vi "Routing Channels.vi"(8 "error in (no error)":errorcluster, 11 "Node Ptr":T1 format="%.0x") -> (0 "error out":errorcluster)   [LabVIEW 2017, in "Routing and Faulting System Explorer.lvlib"]
uses:
  Routing and Faulting System Explorer.lvlib
  <vilib>/NI Veristand/Custom Device API/Custom Device Item Ref.ctl
  Main Page Controls.ctl
  <vilib>/NI VeriStand/Custom Device API/Custom Device API.lvlib
panel:
  out "Version":string
  in  "SHDocVw.IWebBrowser":refnum<k7>(container)
  in  "Description":string
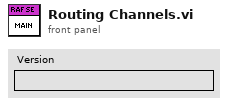
[diagram p1: front panel]
types:
  T1 = typedef "Custom Device API.lvlib/Custom Device Item Ref.ctl" = u64
  T2 = typedef "Routing and Faulting System Explorer.lvlib/Main Page Controls.ctl" = cluster{"Description":refnum<vi>, "Version":refnum<vi>}
  T3 = typedef "Custom Device API.lvlib/Custom Device Commands.ctl" = enum16{"Default", "Item renamed", "Shutdown", "Dynamic button pressed"}
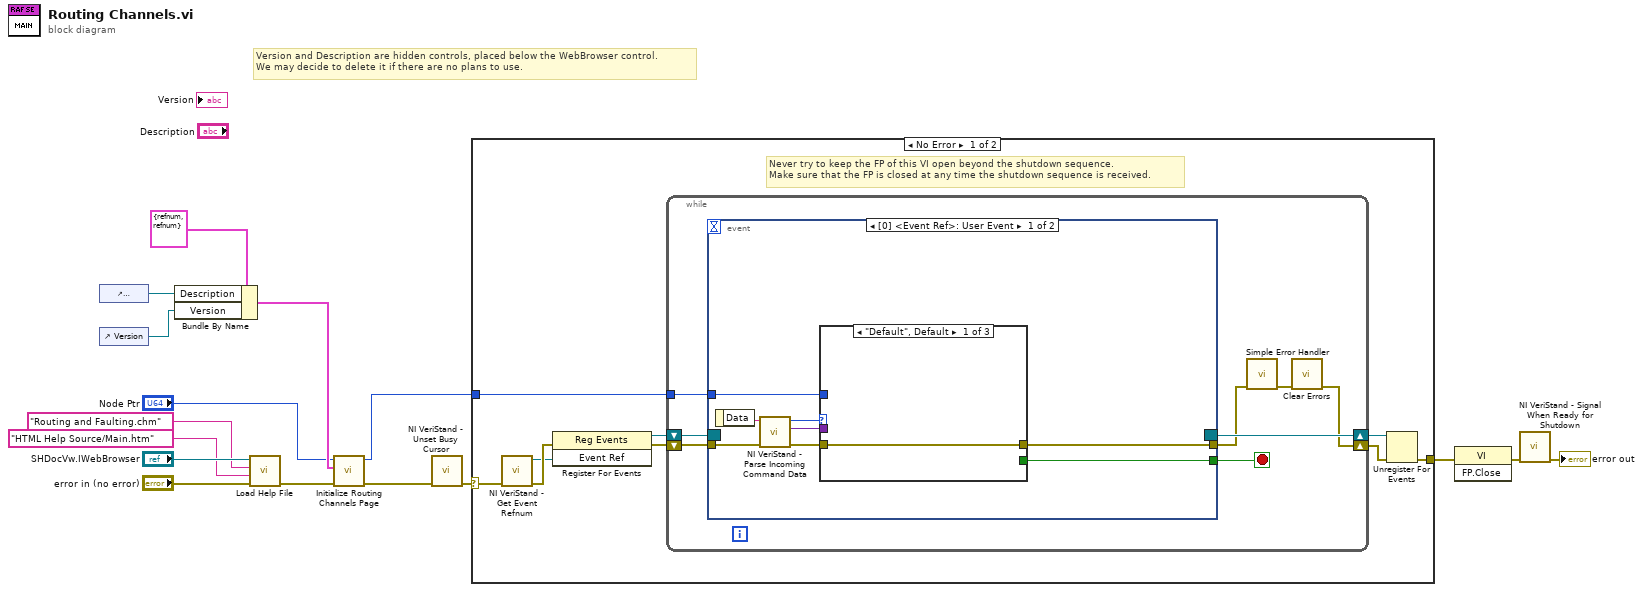
[diagram p0: block diagram]
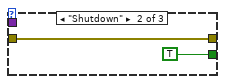
[diagram p2: hidden frame]
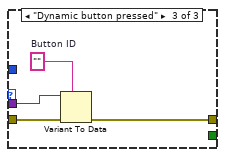
[diagram p3: hidden frame]
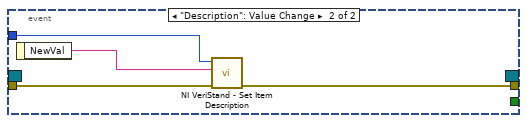
[diagram p4: hidden frame]
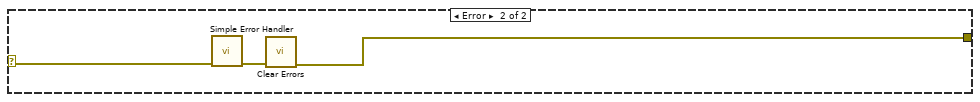
[diagram p5: hidden frame]
diagram:
  # "Version and Description are hidden controls, placed below the WebBrowser control.\nWe may decide to delete it if there are no plans to use."
  n1 = control-ref of="Description"() -> (w7:refnum<vi>)
  n2 = control-ref of="Version"() -> (w6:refnum<vi>)
  n3 = Bundle By Name(cluster=T2 {"Description"=refnum, "Version"=refnum} ("Main Page Controls"), "Description"=w7, "Version"=w6) -> (w5:T2)
  n4 = call "Load Help File.vi"("error in (no error)"="error in (no error)", "HTML File to Load"="HTML Help Source/Main.htm" ("HTML File"), "Main CHM File"="Routing and Faulting.chm" ("CD_CHM_FileName"), "Browser"="SHDocVw.IWebBrowser") -> ("error out"=w4:errorcluster)  [unwired: 7 in]
  n5 = call "Initialize Routing Channels Page.vi"("error in (no error)"=w4, "Main Page Controls"=w5, "Item Ref in"="Node Ptr") -> ("error out"=w3:errorcluster, "Item Ref out"=w1:T1)  [unwired: 7 in]
  n6 = call <vilib>:"NI VeriStand - Unset Busy Cursor.vi"("error in (no error)"=w3) -> ("error out"=w13:errorcluster)  [unwired: 10 out]
  n7 = case shown="No Error" w13 {
    selector: w13 -> [w17 w55]
    tunnel: [w22 w53] -> w16
    tunnel: w1 -> [w18 _]
    frame No Error {
      # "Never try to keep the FP of this VI open beyond the shutdown sequence.\nMake sure that the FP is closed at any time the shutdown sequence is received."
      n8 = call <vilib>:"NI VeriStand - Get Event Refnum.vi"("error in (no error)"=w17) -> ("error out"=w25:errorcluster, "Event Ref"=w21:refnum<user-event>)  [unwired: 9 out]
      n9 = register-events(error in=w25, w21) -> (reference out=w19:refnum<event-registration>, error out=w20:errorcluster)  [unwired: 1 in]
      n10 = while {
        tunnel: w18 -> [w29]
        shift-right: [w26] -> w23
        shift-left: w20 -> [w32]
        shift-right: [w33] -> w24
        shift-left: w19 -> [w31]
        stop <- w30 stop-if-true
        n11 = event shown="[0] <Event Ref>: User Event" {
          selector: w31 -> [_ _]
          dyn-events: [_ _] -> w33
          timeout: _ -> [_ _]
          tunnel: w32 -> [w41 w51]
          tunnel: [w37 _] -> w30
          tunnel: [w36 w50] -> w28
          tunnel: w29 -> [w35 w52]
          event User Event {
            n12 = event-data() -> ("Data"=w40:string)  [unwired: 1 out]
            n13 = call <vilib>:"NI VeriStand - Parse Incoming Command Data.vi"("error in (no error)"=w41, "Incoming data"=w40) -> ("error out"=w39:errorcluster, "Outgoing data"=w34:variant, "Action"=w38:T3)  [unwired: 7 out]
            n14 = case shown="\"Default\", Default" w38 {
              tunnel: w39 -> [w42 w43 w48]
              tunnel: [_ TRUE _] -> w37
              tunnel: [w42 w43 w45] -> w36
              tunnel: w35 -> [_ _ _]
              tunnel: w34 -> [_ _ w47]
              frame "Default", Default {
              }
              frame "Shutdown" {
              }
              frame "Dynamic button pressed" {
                w46 = ""  # Button ID
                n15 = Variant To Data(error in=w48, type=w46, Variant=w47) -> (error out=w45:errorcluster)  [unwired: 1 out]
              }
            }
          }
          event "Description": Value Change {
            n16 = event-data() -> ("NewVal"=w49:string)  [unwired: 1 out]
            n17 = call <vilib>:"NI VeriStand - Set Item Description.vi"("error in (no error)"=w51, "Description"=w49, "Item Ref in"=w52) -> ("error out"=w50:errorcluster)  [unwired: 8 out]
          }
        }
        n18 = call <vilib>:"Simple Error Handler.vi"("error in (no error)"=w28) -> ("error out"=w27:errorcluster)  [unwired: 1 in, 7 out]
        n19 = call <vilib>:"Clear Errors.vi"("error in (no error)"=w27) -> ("error out"=w26:errorcluster)  [unwired: 1 in, 5 out]
      }
      n20 = Unregister For Events(event registration refnum=w24, error in=w23) -> (error out=w22:errorcluster)
    }
    frame Error {
      n21 = call <vilib>:"Simple Error Handler.vi"("error in (no error)"=w55) -> ("error out"=w54:errorcluster)  [unwired: 1 in, 7 out]
      n22 = call <vilib>:"Clear Errors.vi"("error in (no error)"=w54) -> ("error out"=w53:errorcluster)  [unwired: 1 in, 5 out]
    }
  }
  n23 = invoke class="VI" method="FP.Close"(error in=w16) -> (error out=w15:errorcluster)  [unwired: 2 in, 2 out]
  n24 = call <vilib>:"NI VeriStand - Signal When Ready for Shutdown.vi"("error in (no error)"=w15) -> ("error out"=→"error out":errorcluster)  [unwired: 10 out]
